vi "Bristol_WM_SA.vi"() -> ()   [LabVIEW 2012]
uses:
  <vilib>/DAQmx/write.llb/DAQmx Write (Digital 1D Bool NChan 1Samp 1Line).vi
  <vilib>/DAQmx/miscellaneous.llb/DAQmx Fill In Error Info.vi
panel:
  in  "TimeOut":i32=1000
  in  "Lambda":bool
  in  "stop":bool
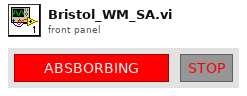
[diagram p1: front panel]
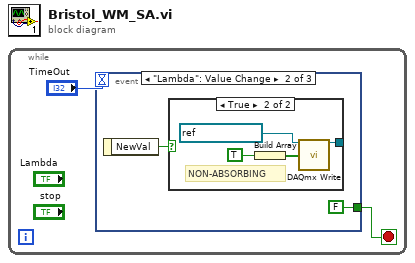
[diagram p0: block diagram]
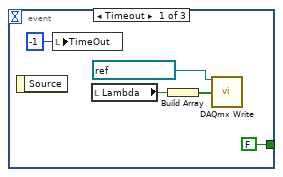
[diagram p2: hidden frame]
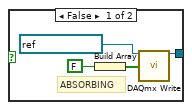
[diagram p3: hidden frame]
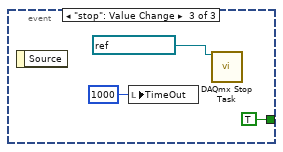
[diagram p4: hidden frame]
diagram:
  n1 = while {
    stop <- w2 stop-if-true
    n2 = event shown="[1] \"Lambda\": Value Change" {
      selector: _ -> [_ _ _]
      dyn-events: _ -> [_ _ _]
      timeout: "TimeOut" -> [_ _ _]
      tunnel: [FALSE ("Boolean") FALSE ("Boolean") TRUE ("Boolean")] -> w2
      event Timeout {
        n3 = event-data() -> ()  [unwired: 1 in, 1 out]
        n4 = local write "TimeOut"(-1 ("TimeOut")) -> ()
        n5 = local read "Lambda"() -> (w3:bool)
        n6 = Build Array(w3) -> (w4:bool[])
        n7 = call-poly <vilib>:"DAQmx Write.vi"("task/channels in"=refnum<k21> "BristolWM", "data"=w4) -> ()  [unwired: 11 in, 3 out]
      }
      event "Lambda": Value Change {
        n8 = event-data() -> ("NewVal"=w9:bool)  [unwired: 1 in]
        n9 = case shown="True" w9 {
          tunnel: [w12 w16] -> _
          frame False {
            # "ABSORBING"
            n10 = Build Array(FALSE ("Boolean")) -> (w10:bool[])
            n11 = call-poly <vilib>:"DAQmx Write.vi"("task/channels in"=refnum<k21> "BristolWM", "data"=w10) -> ("task out"=w12:refnum<k21>)  [unwired: 11 in, 2 out]
          }
          frame True {
            # "NON-ABSORBING"
            n12 = Build Array(TRUE ("Boolean")) -> (w14:bool[])
            n13 = call-poly <vilib>:"DAQmx Write.vi"("task/channels in"=refnum<k21> "BristolWM", "data"=w14) -> ("task out"=w16:refnum<k21>)  [unwired: 11 in, 2 out]
          }
        }
      }
      event "stop": Value Change {
        n14 = event-data() -> ()  [unwired: 1 in, 1 out]
        n15 = local write "TimeOut"(1000 ("TimeOut")) -> ()
        n16 = call <vilib>:"DAQmx Stop Task.vi"("task/channels in"=refnum<k21> "BristolWM") -> ()  [unwired: 13 in, 2 out]
      }
    }
  }
